vi "Build VI HTML.vi"(6 "Destination":path=path "", 7 "Requirement":string="Mustache", 8 "Error In":errorcluster, 11 "VI":path=path "") -> (0 "Error Out":errorcluster)   [LabVIEW 2018, in "Scripts.lvlib"]
uses:
  Scripts.lvlib
  Toolkit/Data/Array/Array.lvclass
  D:/Users/cfield/Code/Field R&D Services/Mustache/LabVIEW/trunk/src/Toolkit/Data/Abstract/Abstract.lvclass
  Toolkit/Data/Map/Map.lvclass
  Toolkit/Data/Map/Support/From String.vi
  Toolkit/Data/Map/Support/From Datum.vi
  Toolkit/Data/Map/Support/From Map Array.vi
  Toolkit/Support/Compile with Data.vi
  Toolkit/Toolkit.lvlib
  <vilib>/Field R&D Services/Labricator/Toolkit/Labricator.lvlib
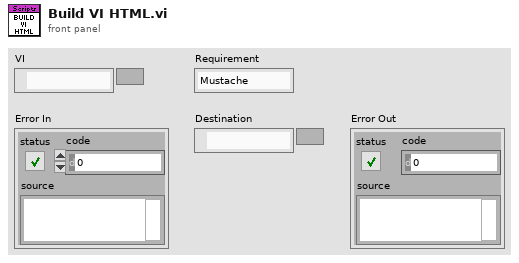
[diagram p1: front panel]
types:
  T1 = enum16{"open", "replace", "create", "open or create", "replace or create", "replace or create with confirmation"}
  T2 = cluster{"Alt":string, "Description":string, "Src":string}[]
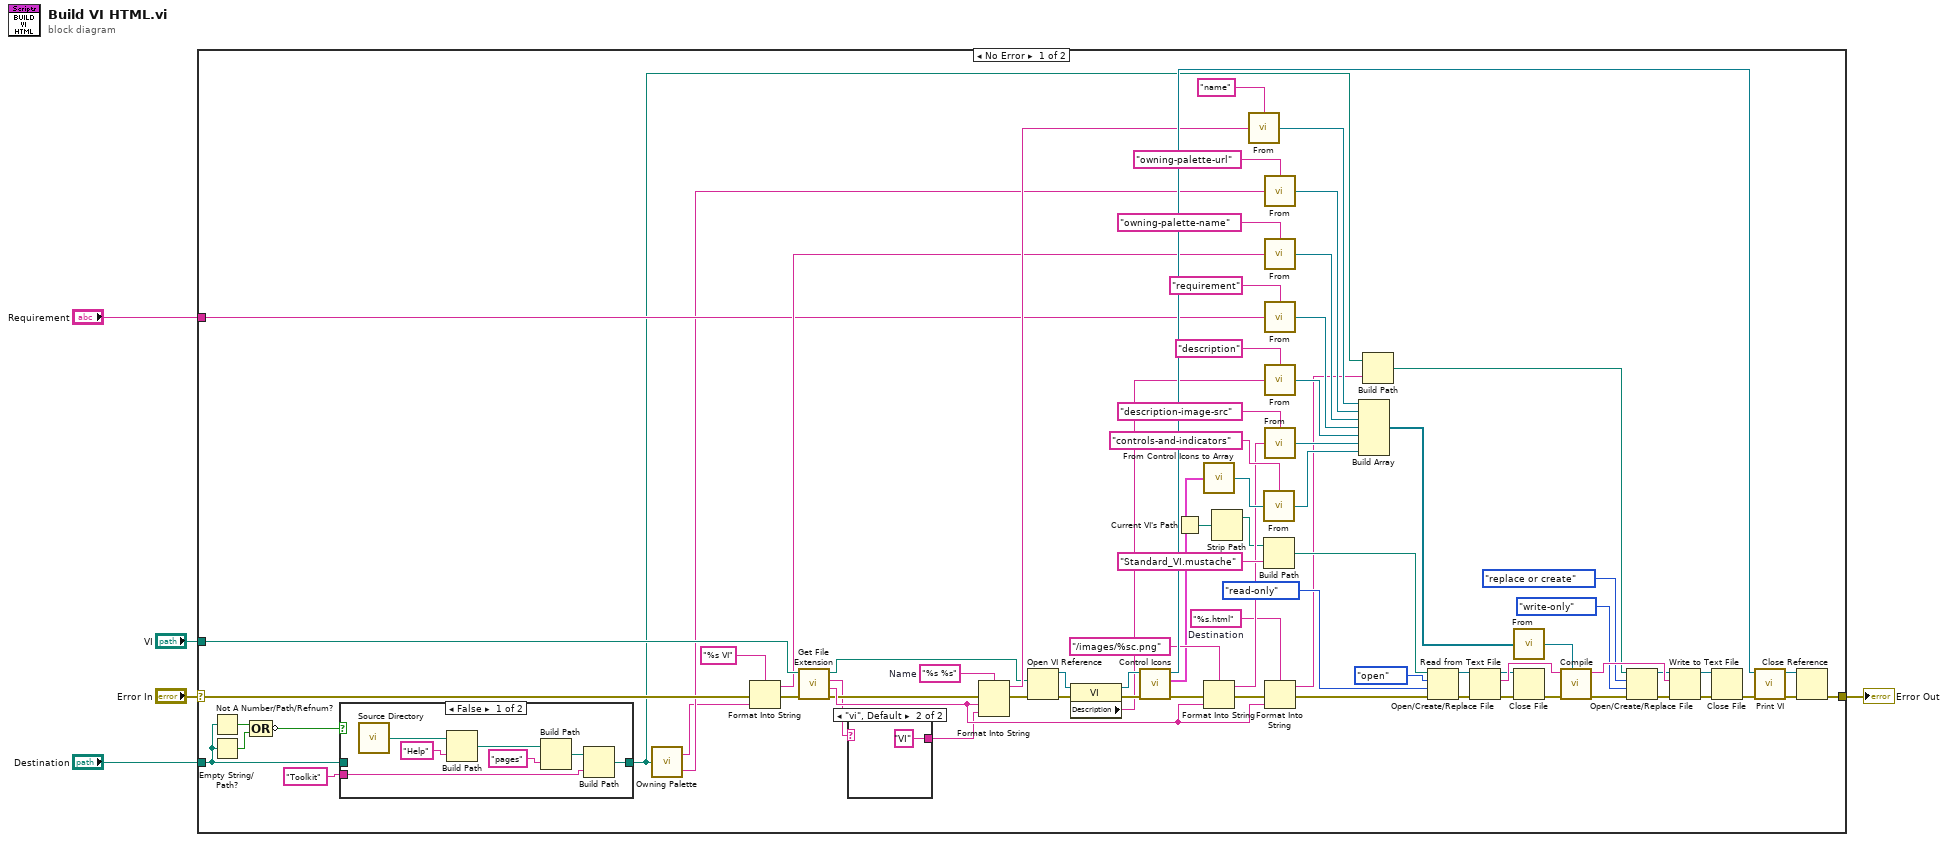
[diagram p0: block diagram]
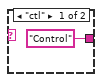
[diagram p3: hidden frame]
diagram:
  n1 = case shown="No Error" "Error In" {
    selector: "Error In" -> [w11 w94]
    tunnel: [w78 w94] -> w5
    tunnel: "VI" -> [w24 _]
    tunnel: "Destination" -> [w17 _]
    tunnel: "Requirement" -> [w12 _]
    frame No Error {
      w27 = "%s %s"  # Name
      w22 = "%s.html"  # Destination
      n2 = Not A Number/Path/Refnum?(number/path/refnum=w17) -> (NaN/Path/Refnum?=w19:bool)
      n3 = Empty String/Path?(string/path=w17) -> (empty?=w20:bool)
      n4 = Compound Arithmetic op=OR(w19, w20) -> (invert w18:bool)
      n5 = case shown="False" w18 {
        tunnel: w17 -> [_ w91]
        tunnel: [w85 w91] -> w9
        tunnel: "Toolkit" ("name or relative path") -> [w84 _]
        frame False {
          n6 = call <vilib>:"Source Directory.vi"() -> ("Source Directory"=w90:path)
          n7 = Build Path(base path=w90, name or relative path="Help") -> (appended path=w88:path)
          n8 = Build Path(base path=w88, name or relative path="pages") -> (appended path=w86:path)
          n9 = Build Path(base path=w86, name or relative path=w84) -> (appended path=w85:path)
        }
        frame True {
        }
      }
      n10 = call "Owning Palette.vi"("Destination"=w9) -> ("Name"=w7:string, "URL"=w8:string)
      n11 = Format Into String(format string="%s VI", error in=w11, w7) -> (resulting string=w13:string, error out=w15:errorcluster)  [unwired: 1 in]
      n12 = call <vilib>:"Get File Extension.vi"("error in (no error)"=w15, "file"=w24) -> ("error out"=w28:errorcluster, "filename without extension"=w80:string, "lowercase file extension"=w26:string, "dup file"=w25:path)  [unwired: 5 in, 1 out]
      n13 = case shown="\"vi\", Default" w26 {
        tunnel: ["Control" "VI"] -> w30
        frame "ctl" {
        }
        frame "vi", Default {
        }
      }
      n14 = Format Into String(format string=w27, error in=w28, w80, w30) -> (resulting string=w32:string, error out=w29:errorcluster)  [unwired: 1 in]
      n15 = Open VI Reference(vi path=w25, error in (no error)=w29) -> (vi reference=w21:refnum<vi>, error out=w33:errorcluster)  [unwired: 4 in]
      n16 = property class="VI"(reference=w21, error in=w33) -> (reference out=w81:refnum<vi>, error out=w70:errorcluster, "Description"=w34:string)
      n17 = call "Control Icons.vi"("Error In"=w70, "VI In"=w81) -> ("Error Out"=w83:errorcluster, "Control Icons"=w6:T2, "VI Out"=w82:refnum<vi>)  [unwired: 7 in]
      n18 = Current VI's Path() -> (path=w42:path)
      n19 = call "From Control Icons to Array.vi"("Control Icons"=w6) -> ("Array"=w76:refnum<class "Array.lvclass">)
      n20 = Format Into String(format string="/images/%sc.png", error in=w83, w80) -> (resulting string=w38:string, error out=w37:errorcluster)  [unwired: 1 in]
      n21 = Strip Path(path=w42) -> (stripped path=w16:path)  [unwired: 1 out]
      n22 = call-poly "From.vi"("Value"=w32, "Key"="name") -> ("Map"=w67:refnum<class "Map.lvclass">)
      n23 = call-poly "From.vi"("Value"=w76, "Key"="controls-and-indicators") -> ("Map"=w64:refnum<class "Map.lvclass">)
      n24 = Build Path(base path=w16, name or relative path="Standard_VI.mustache") -> (appended path=w44:path)
      n25 = call-poly "From.vi"("Value"=w8, "Key"="owning-palette-url") -> ("Map"=w75:refnum<class "Map.lvclass">)
      n26 = call-poly "From.vi"("Value"=w13, "Key"="owning-palette-name") -> ("Map"=w73:refnum<class "Map.lvclass">)
      n27 = call-poly "From.vi"("Value"=w12, "Key"="requirement") -> ("Map"=w71:refnum<class "Map.lvclass">)
      n28 = call-poly "From.vi"("Value"=w34, "Key"="description") -> ("Map"=w66:refnum<class "Map.lvclass">)
      n29 = call-poly "From.vi"("Value"=w38, "Key"="description-image-src") -> ("Map"=w65:refnum<class "Map.lvclass">)
      n30 = Format Into String(format string=w22, error in=w37, w80) -> (resulting string=w23:string, error out=w45:errorcluster)  [unwired: 1 in]
      n31 = Build Array(w67, w75, w73, w71, w66, w65, w64) -> (w68:refnum<class "Map.lvclass">[])
      n32 = Build Path(base path=w9, name or relative path=w23) -> (appended path=w55:path)
      n33 = Open/Create/Replace File(file path (use dialog)=w44, error in=w45, operation (0:open)=T1."open", access (0:read/write)=enum16{"read/write", "read-only", "write-only"}."read-only") -> (refnum out=w48:refnum<file>, error out=w49:errorcluster)  [unwired: 2 in, 1 out]
      n34 = Read from Text File(file (use dialog)=w48, error in=w49) -> (refnum out=w50:refnum<file>, text=w53:string, error out=w51:errorcluster)  [unwired: 2 in, 1 out]
      n35 = call-poly "From.vi"("Maps"=w68) -> ("Map"=w69:refnum<class "Map.lvclass">)  [unwired: 1 in]
      n36 = Close File(refnum=w50, error in=w51) -> (error out=w52:errorcluster)  [unwired: 1 out]
      n37 = call-poly "Compile.vi"("Data"=w69, "Error In"=w52, "Input"=w53) -> ("Error Out"=w54:errorcluster, "Output"=w60:string)  [unwired: 7 in]
      n38 = Open/Create/Replace File(file path (use dialog)=w55, error in=w54, operation (0:open)=T1."replace or create", access (0:read/write)=enum16{"read/write", "read-only", "write-only"}."write-only") -> (refnum out=w58:refnum<file>, error out=w59:errorcluster)  [unwired: 2 in, 1 out]
      n39 = Write to Text File(file (use dialog)=w58, text=w60, error in=w59) -> (refnum out=w61:refnum<file>, error out=w62:errorcluster)  [unwired: 1 in, 1 out]
      n40 = Close File(refnum=w61, error in=w62) -> (error out=w63:errorcluster)  [unwired: 1 out]
      n41 = call "Print VI.vi"("Error In"=w63, "VI In"=w82) -> ("Error Out"=w77:errorcluster, "VI Out"=w79:refnum<vi>)  [unwired: 8 in]
      n42 = Close Reference(reference=w79, error in (no error)=w77) -> (error out=w78:errorcluster)
    }
    frame Error {
    }
  }
  "Error Out" <- w5
